vi "Set CPU Pools.vi"(8 "error in (no error)":errorcluster caption="错误输入（无错误）") -> (0 "error out":errorcluster caption="错误输出", 2 "Processor Assignment":i32 caption="处理器分配")   [LabVIEW 2013]
uses:
  <vilib>/Utility/RT CPU pool selections.ctl
  <vilib>/NI_Real-Time Target Support.lvlib
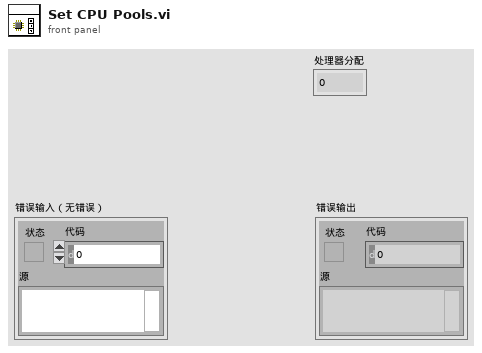
[diagram p1: front panel]
types:
  T1 = typedef "NI_Real-Time Target Support.lvlib/RT CPU pool selections.ctl" = enum16{"System & Timed Structures", "System", "Timed Structures", "Reserved"}
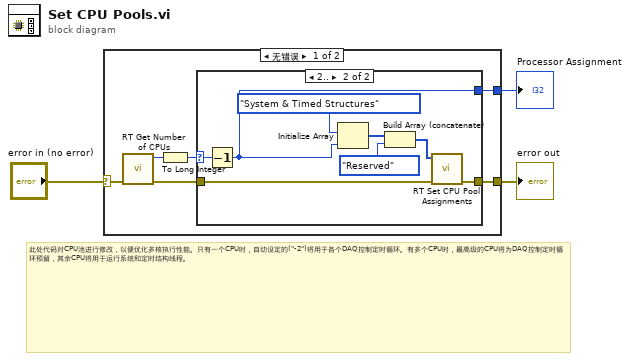
[diagram p0: block diagram]
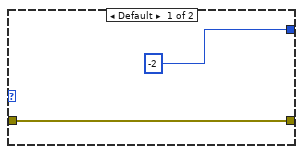
[diagram p2: hidden frame]
diagram:
  # "此处代码对CPU池进行修改，以便优化多核执行性能。只有一个CPU时，自动设定的(\"-2\")将用于各个DAQ控制定时循环。有多个CPU时，最高级的CPU将为DAQ控制定时循环预留，其余CPU将用于运行系统和定时结构线程。"
  n1 = case shown="无错误" "error in (no error)" {
    selector: "error in (no error)" -> [w7 w20]
    tunnel: [w8 w20] -> w3
    tunnel: [w5 _] -> w1
    frame No Error {
      n2 = call <vilib>:"RT Get Number of CPUs.vi"("error in (no error)"=w7) -> ("error out"=w9:errorcluster, "# of CPUs"=w6:u32)  [unwired: 9 in]
      n3 = To Long Integer(number=w6) -> (32bit integer=w4:i32)
      n4 = case shown="2.." w4 {
        selector: w4 -> [_ w13]
        tunnel: w9 -> [w11 w19]
        tunnel: [w11 w18] -> w8
        tunnel: [-2 ("# of CPUs") w12] -> w5
        frame Default {
        }
        frame 2.. {
          n5 = Decrement(x=w13) -> (x-1=w12:i32)
          n6 = Initialize Array(RT_CPU_pool_selections."System & Timed Structures" ("Enum"), w12) -> (w16:T1[])
          n7 = Build Array (concatenate)(w16, RT_CPU_pool_selections."Reserved" ("Enum")) -> (w14:T1[])
          n8 = call <vilib>:"RT Set CPU Pool Assignments.vi"("error in (no error)"=w19, "CPU pools"=w14) -> ("error out"=w18:errorcluster)  [unwired: 6 in, 3 out]
        }
      }
    }
    frame Error {
    }
  }
  "error out" <- w3
  "Processor Assignment" <- w1
